vi "Launch Terminal.vi"(8 "error in (no error)":errorcluster, 11 "Manager in":refnum<class "Manager.lvclass">) -> (0 "error out":errorcluster, 3 "Manager out":refnum<class "Manager.lvclass">)   [LabVIEW 2025, in "Manager.lvlib" / "Manager.lvclass"]
uses:
  Manager.lvclass
  Manager.lvclass/Manager.ctl
  <vilib>/ActorFramework/Actor/Actor.lvclass
  UI VISA Terminal/UI VISA Terminal/UI VISA Terminal.lvclass
  C:/Program Files/National Instruments/LabVIEW 2025/vi.lib/ActorFramework/Actor/Actor.lvclass
  C:/Users/juan_/Desktop/Lab it Studio/Public/Sesiones/Sesiones/Sesion [11] 14 Julio 2025/AF VISA Terminal/UI VISA Terminal/UI VISA Terminal/UI VISA Terminal.lvclass
  C:/Users/juan_/Desktop/Lab it Studio/Public/Sesiones/Sesiones/Sesion [11] 14 Julio 2025/AF VISA Terminal/Manager/Manager/Manager.lvclass
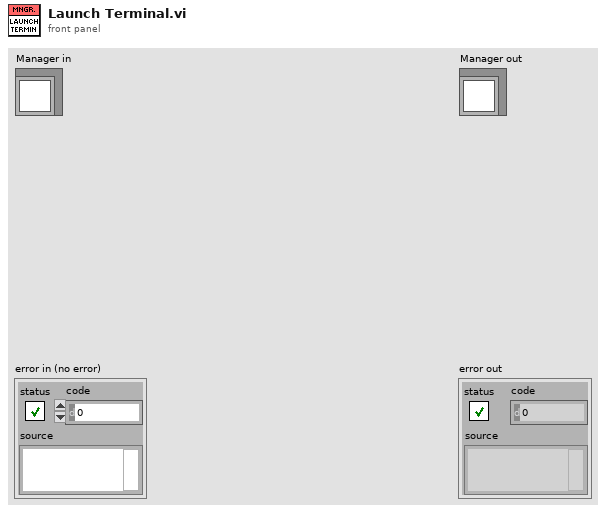
[diagram p1: front panel]
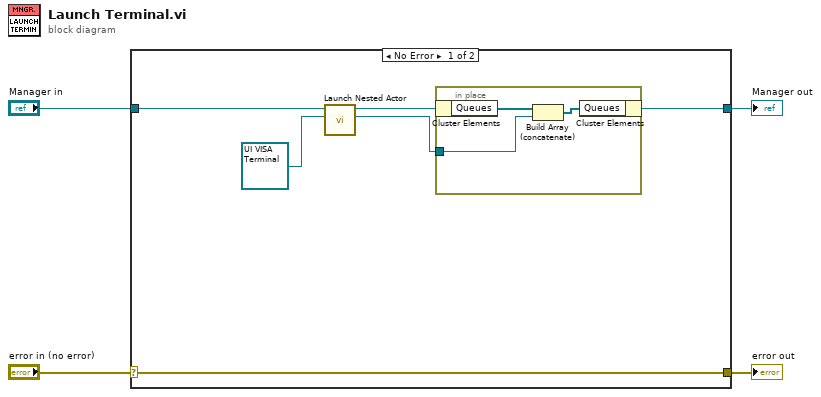
[diagram p0: block diagram]
diagram:
  n1 = case shown="No Error" "error in (no error)" {
    selector: "error in (no error)" -> [w10 w15]
    tunnel: [w10 w15] -> w3
    tunnel: [w5 w14] -> w1
    tunnel: "Manager in" -> [w9 w14]
    frame No Error {
      n2 = call <vilib>:"Launch Nested Actor.vi"("Nested Actor"=refnum<class "UI VISA Terminal.lvclass"> refnum ("UI VISA Terminal.lvlib:UI VISA Terminal.lvclass"), "Caller Actor in"=w9) -> ("Nested Actor's Enqueuer"=w6:refnum<class "Message Enqueuer.lvclass">, "Caller Actor out"=w7:refnum<class "Manager.lvclass">)  [unwired: 7 in, 1 out]
      n3 = in-place {
        in-place-border: w6 -> [w12]
        n4 = in-place-cluster #1(w7) -> ("Queues"=w13:refnum<class "Message Enqueuer.lvclass">[])
        n5 = Build Array (concatenate)(w13, w12) -> (w11:refnum<class "Message Enqueuer.lvclass">[])
        n6 = in-place-cluster #1("Queues"=w11) -> (w5:refnum<class "Manager.lvclass">)
      }
    }
    frame Error {
    }
  }
  "error out" <- w3
  "Manager out" <- w1
